vi "SS Read 3.vi"(8 "error in (no error)":errorcluster, 10 "Number of Bytes to Read":i32, 11 "FPGA VI Reference in":T1) -> (0 "error out":errorcluster, 2 "Data":string, 3 "FPGA VI Reference out":T1)   [LabVIEW 2009]
uses:
  SS FPGA VI Ref.ctl
  <vilib>/rvi/interface/nirviMethod/nirviMethod.xnode
  FPGA Bitfiles/Q_IGVC_2010.lvproj_FPGA Target_GPS diagnostic.vi.lvbitx
  <vilib>/LabVIEW Targets/FPGA/RIO/nirio_HostInterface/nirio_WaitOnIRQ.vi
  <vilib>/RVI Host/nirviSupport.llb/nirviErrorClusterFromErrorCode.vi
  <vilib>/rvi/interface/common/niFpgaNodeNameForErrorReporting.ctl
  <vilib>/rvi/errors/niLvFpgaWhatHappensToTopLevelVI.ctl
  <vilib>/rvi/errors/niLvFpgaAdjustHostInterfaceError.vi
  <vilib>/Utility/error.llb/Error Cluster From Error Code.vi
  <vilib>/rvi/interface/nirviReadWriteControl/nirviReadWriteControl.xnode
  NiRioSrv.dll
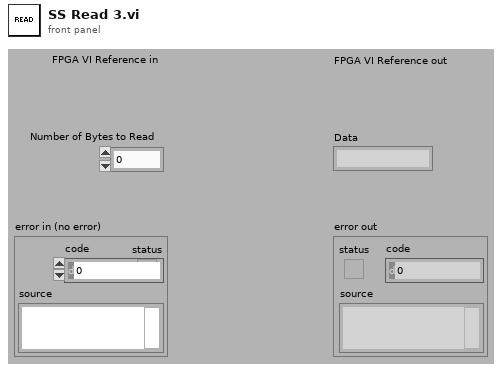
[diagram p1: front panel]
types:
  T1 = typedef "SS FPGA VI Ref.ctl" = refnum<k20>
  T2 = typedef "niFpgaNodeNameForErrorReporting.ctl" = enum16{"Open FPGA VI Reference", "Read/Write Control", "Invoke Method: Abort", "Invoke Method: Acknowledge IRQ", "Invoke Method: Download", "Invoke Method: FIFO.Configure", "Invoke Method: FIFO.Read", "Invoke Method: FIFO.Start", "Invoke Method: FIFO.Stop", "Invoke Method: FIFO.Write", "Invoke Method: Reset", "Invoke Method: Run", "Invoke Method: Wait on IRQ", "Close FPGA VI Reference"}
  T3 = typedef "niLvFpgaWhatHappensToTopLevelVI.ctl" = enum16{"top level VI scripted behind XNode", "top level VI inlined behind XNode"}
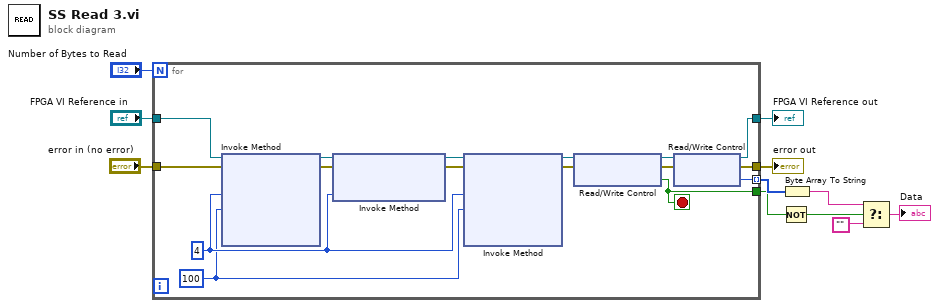
[diagram p0: block diagram]
diagram:
  n1 = for {
    N: "Number of Bytes to Read" -> [_]
    tunnel: "FPGA VI Reference in" -> [w27]
    tunnel: [w22] -> w10
    tunnel: [w21] -> w9
    tunnel: "error in (no error)" -> [w20]
    tunnel: [w19] -> w7 mode=indexing
    tunnel: [w12] -> w2
    stop <- w12 stop-if-true
    w17 = 100 ("Timeout (ms)")
    w18 = 4 ("IRQ Number(s)")
    n2 = xnode "Invoke Method"("FPGA VI Reference In"=w27, "error in"=w20, "IRQ Number(s)"=w18, "Timeout (ms)"=w17) -> ("FPGA VI Reference Out"=w26:T1, "error out"=w25:errorcluster)  [unwired: 2 out]
    n3 = xnode "Invoke Method"("FPGA VI Reference In"=w26, "error in"=w25, "IRQ Number(s)"=w18) -> ("FPGA VI Reference Out"=w24:T1, "error out"=w23:errorcluster)
    n4 = xnode "Invoke Method"("FPGA VI Reference In"=w24, "error in"=w23, "IRQ Number(s)"=w18, "Timeout (ms)"=w17) -> ("FPGA VI Reference Out"=w16:T1, "error out"=w15:errorcluster)  [unwired: 2 out]
    n5 = xnode "Read/Write Control"("FPGA VI Reference In"=w16, "error in"=w15) -> ("FPGA VI Reference Out"=w13:T1, "error out"=w14:errorcluster, "SS Timeout 3"=w12:bool)
    n6 = xnode "Read/Write Control"("FPGA VI Reference In"=w13, "error in"=w14) -> ("FPGA VI Reference Out"=w22:T1, "error out"=w21:errorcluster, "SS Data 3"=w19:u8)
  }
  "FPGA VI Reference out" <- w10
  "error out" <- w9
  n7 = Not(x=w2) -> (.not. x?=w1:bool)
  n8 = Byte Array To String(unsigned byte array=w7) -> (string=w4:string)
  n9 = Select(t=w4, s=w1, f="") -> (s? t:f=→"Data":string)
